vi "Configure Baud Rate.vi"(8 "error in (no error)":errorcluster, 9 "Baud rate (57600 bps)":T1=34 items=["1,000,000 bps"=1, "500,000 bps"=3, "400,000 bps"=4, "250,000 bps"=7, "200,000 bps"=9, "115200 bps"=16, "57600 bps"=34, "19200 bps"=103, "9600 bps"=207], 10 "Motor ID (0)":u8, 11 "VISA resource name":refnum<visa-resource-name>) -> (0 "error out":errorcluster, 3 "VISA resource name out":refnum<visa-resource-name>)   [LabVIEW 2016, in "Dynamixel Motor.lvlib"]
doc: "Sets the motor's baud rate. The motor will automatically \"reboot\" and respond to commands sent using the new baud rate."
uses:
  Dynamixel Motor.lvlib
  Motor Operation/Low Level/Baud Setting.ctl
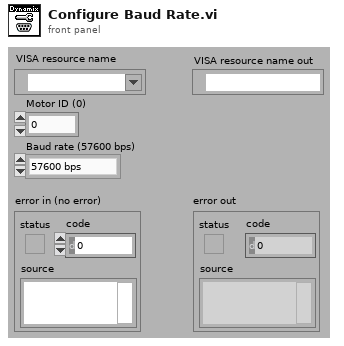
[diagram p1: front panel]
types:
  T1 = typedef "Dynamixel Motor.lvlib/Baud Setting.ctl" = u8
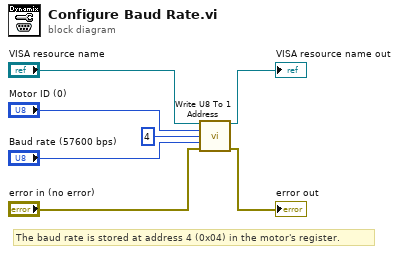
[diagram p0: block diagram]
diagram:
  # "The baud rate is stored at address 4 (0x04) in the motor's register."
  n1 = call "Write U8 To 1 Address.vi"("VISA resource name"="VISA resource name", "Motor ID (0)"="Motor ID (0)", "Address number (0)"=u8 4 ("Address"), "Parameter (0)"="Baud rate (57600 bps)", "error in (no error)"="error in (no error)") -> ("VISA resource name out"=→"VISA resource name out":refnum<visa-resource-name>, "error out"=→"error out":errorcluster)  [unwired: 9 in]
